vi "Compute Xi.vi"(8 "Beta":dbl[][](array[numeric]), 9 "Alpha":dbl[][](array[numeric]), 10 "Observed sequence O":i32[](array[numeric]), 11 "HMM Cluster":T1) -> (3 "Xi":dbl[][][](array[numeric]))   [LabVIEW 2014, in "HMM.lvlib"]
doc: "Calculates the value of Xi."
uses:
  HMM.lvlib
  Control/HMM Cluster.ctl
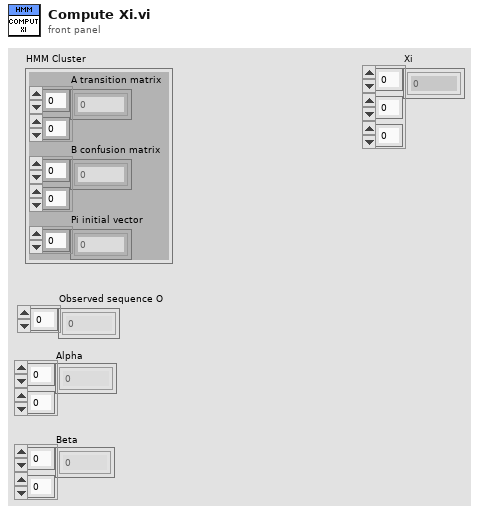
[diagram p1: front panel]
types:
  T1 = typedef "HMM.lvlib/HMM Cluster.ctl" = cluster{"A transition matrix":dbl[][], "B confusion matrix":dbl[][], "Pi initial vector":dbl[]}
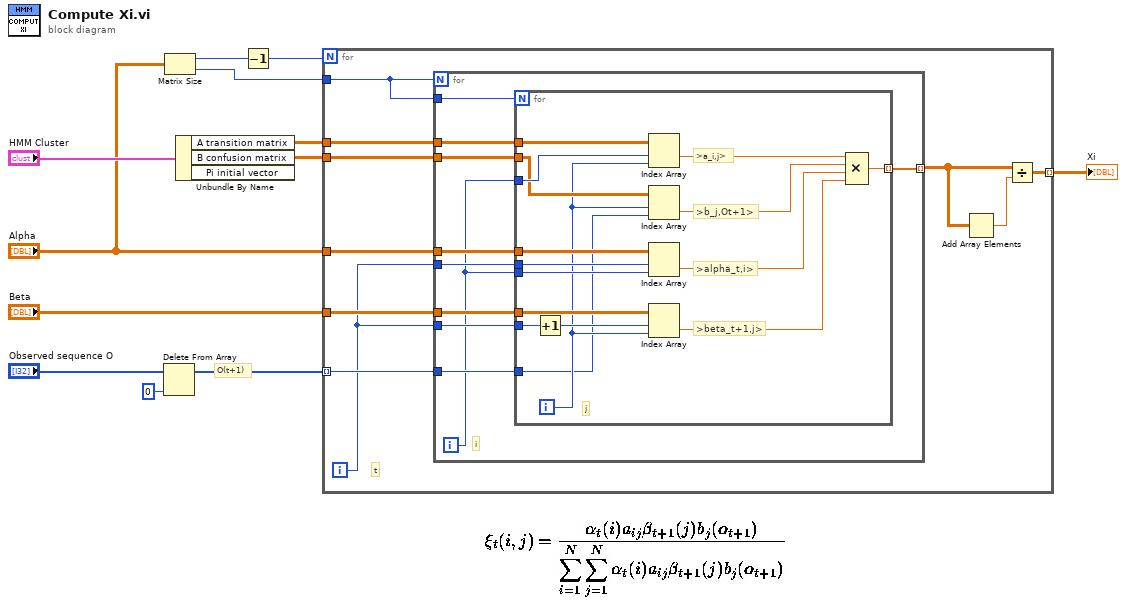
[diagram p0: block diagram]
diagram:
  # "O(t+1)"
  n1 = Delete From Array(array="Observed sequence O", index=0) -> (array with subset deleted=w6:i32[])  [unwired: 1 in, 1 out]
  n2 = Matrix Size(0:"Alpha") -> (1:w12:i32, 2:w7:i32)
  n3 = Unbundle By Name("HMM Cluster") -> ("A transition matrix"=w10:dbl[][], "B confusion matrix"=w9:dbl[][])  [unwired: 1 out]
  n4 = Decrement(x=w12) -> (x-1=w11:i32)
  n5 = for {
    N: w11 -> [_]
    tunnel: "Alpha" -> [w22]
    tunnel: "Beta" -> [w21]
    tunnel: w6 -> [w20] mode=indexing
    tunnel: w10 -> [w18]
    tunnel: w9 -> [w17]
    tunnel: [w14] -> w8 mode=indexing
    tunnel: w7 -> [w13]
    i -> [w19]
    # "t"
    n6 = for {
      N: w13 -> [_]
      tunnel: w22 -> [w32]
      tunnel: w21 -> [w31]
      tunnel: w20 -> [w30]
      tunnel: w19 -> [w29]
      tunnel: w19 -> [w28]
      tunnel: w18 -> [w27]
      tunnel: w17 -> [w26]
      tunnel: [w24] -> w16 mode=indexing
      tunnel: w13 -> [w23]
      i -> [w25]
      # "i"
      n7 = for {
        N: w23 -> [_]
        tunnel: w32 -> [w48]
        tunnel: w31 -> [w47]
        tunnel: w30 -> [w33]
        tunnel: w29 -> [w46]
        tunnel: w25 -> [w45]
        tunnel: w28 -> [w44]
        tunnel: w27 -> [w42]
        tunnel: w26 -> [w40]
        tunnel: w25 -> [w41]
        tunnel: [w34] -> w24 mode=indexing
        i -> [w39]
        # "j"
        # ">beta_t+1,j>"
        # ">alpha_t,i>"
        # ">b_j,Ot+1>"
        # ">a_i,j>"
        n8 = Increment(x=w44) -> (x+1=w43:i32)
        n9 = Index Array(array=w42, index (row)=w41, index (col)=w39) -> (element=w38:dbl)
        n10 = Index Array(array=w40, index (row)=w39, index (col)=w33) -> (element=w37:dbl)
        n11 = Index Array(array=w48, index (row)=w46, index (col)=w45) -> (element=w36:dbl)
        n12 = Index Array(array=w47, index (row)=w43, index (col)=w39) -> (element=w35:dbl)
        n13 = Compound Arithmetic op=MULTIPLY(w38, w37, w36, w35) -> (w34:dbl)
      }
    }
    n14 = Add Array Elements(numeric array=w16) -> (sum=w15:dbl)
    n15 = Divide(x=w16, y=w15) -> (x/y=w14:dbl[][])
  }
  "Xi" <- w8
